vi "ADC GUI Disable types.vi"(5 "Tab ref":refnum<vi>, 7 "Enum ref":refnum<vi>, 8 "error in (no error)":errorcluster) -> (0 "error out":errorcluster)   [LabVIEW 2020]
doc: "Disable digitizer types according conditional symbols w_niscope and w_visa."
uses:
  ADC Type.ctl
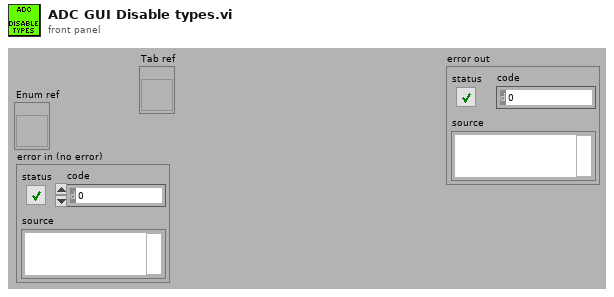
[diagram p1: front panel]
types:
  T1 = typedef "ADC Type.ctl" = enum16{"niScope", "3458A", "DirectSound DLL", "Keysight DSO", "cDAQ ADC", "CMI ADS127L21", "dummy"}
  T2 = enum32{"Page Enabled", "Page Disabled", "Page Disabled & Grayed"}
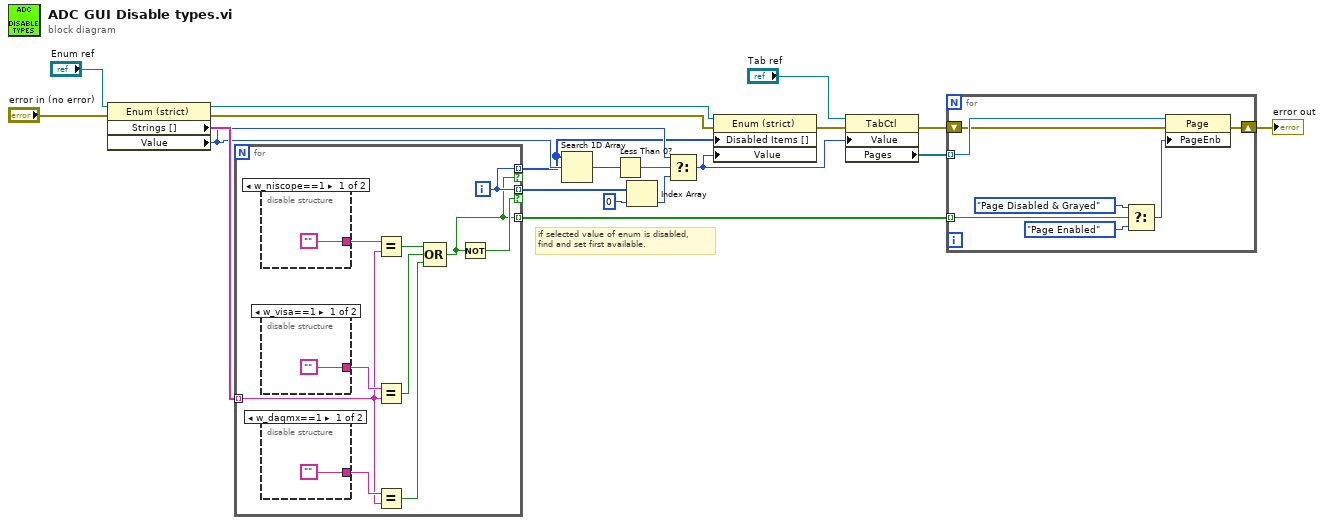
[diagram p0: block diagram]
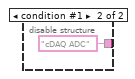
[diagram p2: hidden frame]
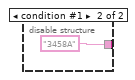
[diagram p3: hidden frame]
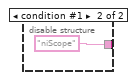
[diagram p4: hidden frame]
diagram:
  # "if selected value of enum is disabled,\nfind and set first available."
  n1 = property class="Enum (strict)"(reference="Enum ref", error in="error in (no error)") -> (reference out=w17:refnum<vi>, error out=w16:errorcluster, "Strings []"=w18:string[], "Value"=w12:T1)
  n2 = for {
    tunnel: w18 -> [w21] mode=indexing
    tunnel: [w24] -> w8 mode=indexing if=w23
    tunnel: [w24] -> w11 mode=indexing if=w25
    tunnel: [w23] -> w5 mode=indexing
    i -> [w24]
    n3 = disable-structure shown="w_niscope==1" {
      disable-tunnel: ["" "niScope"] -> w29
      frame condition #0 (active) {
      }
      frame condition #1 {
      }
    }
    n4 = disable-structure shown="w_visa==1" {
      disable-tunnel: ["" "3458A"] -> w28
      frame condition #0 (active) {
      }
      frame condition #1 {
      }
    }
    n5 = disable-structure shown="w_daqmx==1" {
      disable-tunnel: ["" "cDAQ ADC"] -> w22
      frame condition #0 (active) {
      }
      frame condition #1 {
      }
    }
    n6 = Equal?(x=w29, y=w21) -> (x = y?=w26:bool)
    n7 = Equal?(x=w28, y=w21) -> (x = y?=w27:bool)
    n8 = Equal?(x=w22, y=w21) -> (x = y?=w20:bool)
    n9 = Compound Arithmetic op=OR(w26, w27, w20) -> (w23:bool)
    n10 = Not(x=w23) -> (.not. x?=w25:bool)
  }
  n11 = Search 1D Array(1D array=w8, element=w12) -> (index of element=w14:i32)  [unwired: 1 in]
  n12 = Less Than 0?(x=w14) -> (x < 0?=w13:bool)
  n13 = Index Array(array=w11, index=u16 0) -> (element=w9:i32)
  n14 = Select(t=w12, s=w13, f=w9) -> (s? t:f=w7:i32)
  n15 = property class="Enum (strict)"(reference=w17, error in=w16, "Disabled Items []"=w8, "Value"=w7) -> (error out=w4:errorcluster)  [unwired: 1 out]
  n16 = property class="TabCtl"(reference="Tab ref", error in=w4, "Value"=w7) -> (error out=w3:errorcluster, "Pages"=w6:refnum<vi>[])  [unwired: 1 out]
  n17 = for {
    tunnel: w6 -> [w42] mode=indexing
    tunnel: w5 -> [w38] mode=indexing
    shift-right: [w36] -> w2
    shift-left: w3 -> [w37]
    n18 = Select(t=T2."Page Disabled & Grayed" ("Page Enabled State"), s=w38, f=T2."Page Enabled" ("Page Enabled State")) -> (s? t:f=w39:T2)
    n19 = property class="Page"(reference=w42, error in=w37, "PageEnb"=w39) -> (error out=w36:errorcluster)  [unwired: 1 out]
  }
  "error out" <- w2
